vi "Configure Master Controller.vi"(8 "error in (no error)":errorcluster, 11 "Master Controller in":refnum<class "Master Controller.lvclass">) -> (0 "error out":errorcluster, 3 "Master Controller out":refnum<class "Master Controller.lvclass">)   [LabVIEW 2015, in "Master Controller Core.lvlib" / "Master Controller.lvclass"]
doc: "This VI reads the EMS-config.ini file in the Confiuguration folder in the Application Directory and parses it for locations for device configuration files and logs."
uses:
  Master Controller.lvclass
  Master Controller.lvclass/Master Controller.ctl
  <vilib>/Utility/config.llb/Read Key (String).vi
  <vilib>/Utility/config.llb/NI_LVConfig.lvlib
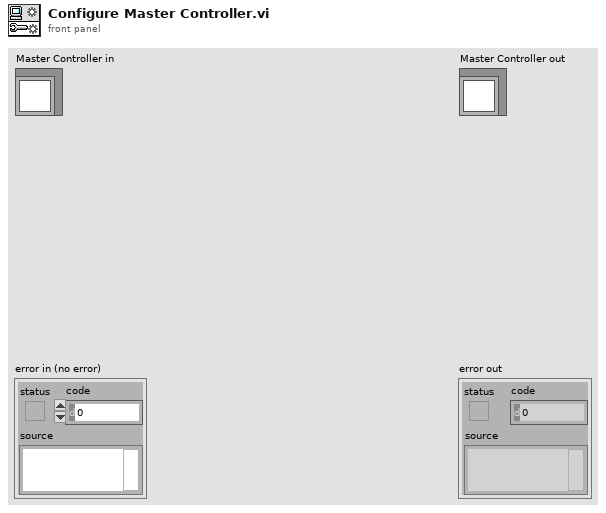
[diagram p1: front panel]
types:
  T1 = typedef "NI_LVConfig.lvlib/Config Data RefNum.ctl" = refnum<k1>
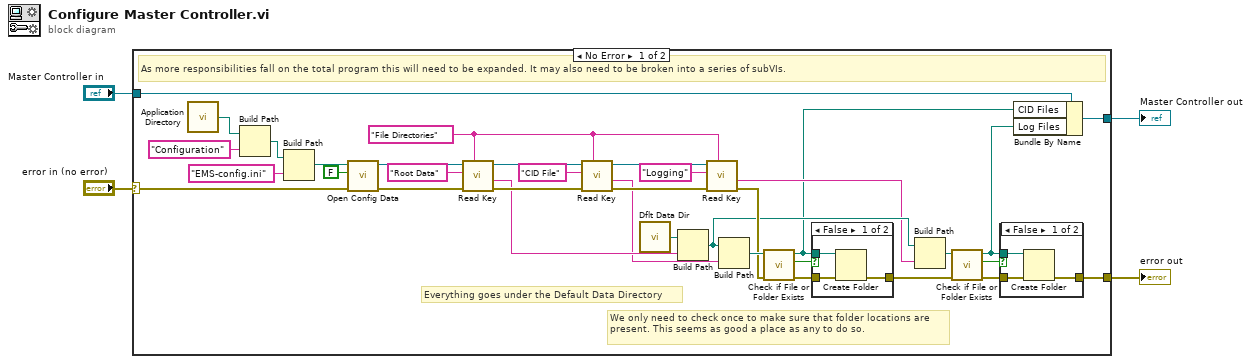
[diagram p0: block diagram]
diagram:
  n1 = case shown="No Error" "error in (no error)" {
    selector: "error in (no error)" -> [w33 w49]
    tunnel: [w5 w49] -> w3
    tunnel: [w8 w48] -> w1
    tunnel: "Master Controller in" -> [w39 w48]
    frame No Error {
      w22 = "File Directories" ("section")
      # "Everything goes under the Default Data Directory"
      # "We only need to check once to make sure that folder locations are present. This seems as good a place as any to do so."
      # "As more responsibilities fall on the total program this will need to be expanded. It may also need to be broken into a series of subVIs."
      n2 = call <vilib>:"Application Directory.vi"() -> ("Application Directory"=w37:path)
      n3 = Build Path(base path=w37, name or relative path="Configuration") -> (appended path=w36:path)
      n4 = Build Path(base path=w36, name or relative path="EMS-config.ini") -> (appended path=w34:path)
      n5 = call <vilib>:"Open Config Data.vi"("error in (no error)"=w33, "create file if necessary (T)"=FALSE, "configuration file path"=w34) -> ("error out"=w30:errorcluster, "refnum"=w31:T1)  [unwired: 6 in, 1 out]
      n6 = call-poly <vilib>:"Read Key.vi"("section"=w22, "error in (no error)"=w30, "key"="Root Data", "refnum"=w31) -> ("error out"=w27:errorcluster, "value"=w17:string, "refnum out"=w28:T1)  [unwired: 4 in, 1 out]
      n7 = call-poly <vilib>:"Read Key.vi"("section"=w22, "error in (no error)"=w27, "key"="CID File", "refnum"=w28) -> ("error out"=w24:errorcluster, "value"=w16:string, "refnum out"=w25:T1)  [unwired: 4 in, 1 out]
      n8 = call <vilib>:"Dflt Data Dir.vi"() -> ("App:Default Data Directory"=w18:path)
      n9 = Build Path(base path=w18, name or relative path=w17) -> (appended path=w10:path)
      n10 = call-poly <vilib>:"Read Key.vi"("section"=w22, "error in (no error)"=w24, "key"="Logging", "refnum"=w25) -> ("error out"=w15:errorcluster, "value"=w9:string)  [unwired: 4 in, 2 out]
      n11 = Build Path(base path=w10, name or relative path=w16) -> (appended path=w19:path)
      n12 = call <vilib>:"Check if File or Folder Exists.vi"("error in (no error)"=w15, "path"=w19) -> ("error out"=w21:errorcluster, "file or folder exists?"=w20:bool, "dup path"=w7:path)  [unwired: 7 in]
      n13 = case shown="False" w20 {
        tunnel: w7 -> [w46 _]
        tunnel: w21 -> [w45 w47]
        tunnel: [w44 w47] -> w11
        frame False {
          n14 = Create Folder(path (use dialog)=w46, error in=w45) -> (error out=w44:errorcluster)  [unwired: 1 in, 2 out]
        }
        frame True {
        }
      }
      n15 = Build Path(base path=w10, name or relative path=w9) -> (appended path=w14:path)
      n16 = call <vilib>:"Check if File or Folder Exists.vi"("error in (no error)"=w11, "path"=w14) -> ("error out"=w12:errorcluster, "file or folder exists?"=w13:bool, "dup path"=w6:path)  [unwired: 7 in]
      n17 = case shown="False" w13 {
        tunnel: w6 -> [w42 _]
        tunnel: w12 -> [w41 w43]
        tunnel: [w40 w43] -> w5
        frame False {
          n18 = Create Folder(path (use dialog)=w42, error in=w41) -> (error out=w40:errorcluster)  [unwired: 1 in, 2 out]
        }
        frame True {
        }
      }
      n19 = Bundle By Name(cluster=w39, "CID Files"=w7, "Log Files"=w6) -> (w8:refnum<class "Master Controller.lvclass">)
    }
    frame Error {
    }
  }
  "error out" <- w3
  "Master Controller out" <- w1
